vi "Configure Operating Mode.vi"(0 "VISA resource name":refnum<visa-resource-name>, 5 "Operating Mode (0: AC Source)":u16(ring) items=["AC Source", "IEC"], 11 "error in (no error)":errorcluster) -> (4 "VISA resource name out":refnum<visa-resource-name>, 15 "error out":errorcluster)   [LabVIEW 2020, in "Agilent 681x Series.lvlib"]
doc: "Configures the operating mode of the instrument.\n\nNote:\nThis VI is only applicable for Agilent/Keysight 6812B, 6813B and 6843A."
uses:
  <instrlib>/Agilent 681x Series/Agilent 681x Series.lvlib
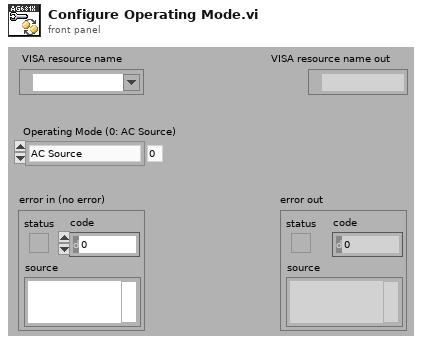
[diagram p1: front panel]
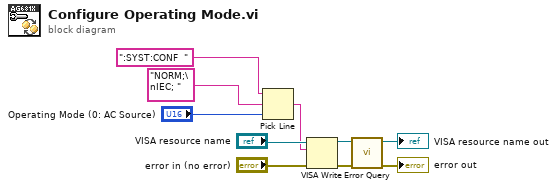
[diagram p0: block diagram]
diagram:
  n1 = Pick Line(string ("")=":SYST:CONF  ", multi-line string="NORM;\nIEC; ", line index="Operating Mode (0: AC Source)") -> (output string=w1:string)
  n2 = VISA Write(VISA resource name="VISA resource name", write buffer=w1, error in (no error)="error in (no error)") -> (VISA resource name out=w8:refnum<visa-resource-name>, error out=w7:errorcluster)  [unwired: 1 out]
  n3 = call <instrlib>:"Error Query.vi"("error in (no error)"=w7, "VISA resource name"=w8) -> ("error out"=→"error out":errorcluster, "VISA resource name out"=→"VISA resource name out":refnum<visa-resource-name>)  [unwired: 6 in, 2 out]
